vi "LaunchProgressBar.vi"(4 "error in":errorcluster, 5 "Title":string, 6 "MaxRange":i32) -> (0 "error out":errorcluster, 3 "reference out":refnum<vi>)   [LabVIEW 2018]
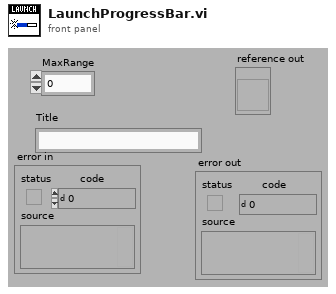
[diagram p1: front panel]
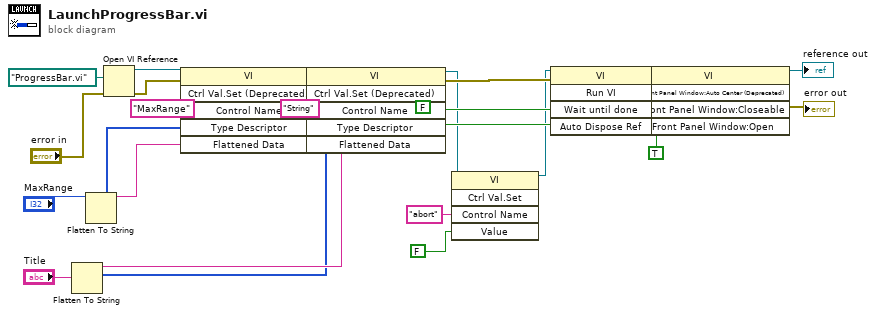
[diagram p0: block diagram]
diagram:
  w5 = FALSE ("Wait until done")
  w23 = TRUE
  n1 = Flatten To String(anything="Title") -> (data string=w12:string, type string=w11:i16[])  [unwired: 3 in, 1 out]
  n2 = Flatten To String(anything="MaxRange") -> (data string=w17:string, type string=w18:i16[])  [unwired: 3 in, 1 out]
  n3 = Open VI Reference(vi path=path "ProgressBar.vi", error in (no error)="error in") -> (vi reference=w20:refnum<vi>, error out=w15:errorcluster)  [unwired: 4 in]
  n4 = invoke class="VI" method="Ctrl Val.Set (Deprecated)"(reference=w20, error in=w15, "Control Name"="MaxRange", "Type Descriptor"=w18, "Flattened Data"=w17) -> (reference out=w14:refnum<vi>, error out=w13:errorcluster)  [unwired: 1 in, 4 out]
  n5 = invoke class="VI" method="Ctrl Val.Set (Deprecated)"(reference=w14, error in=w13, "Control Name"="String", "Type Descriptor"=w11, "Flattened Data"=w12) -> (reference out=w4:refnum<vi>, error out=w8:errorcluster)  [unwired: 1 in, 4 out]
  n6 = invoke class="VI" method="Ctrl Val.Set"(reference=w4, "Control Name"="abort", "Value"=FALSE) -> (reference out=w3:refnum<vi>)  [unwired: 2 in, 4 out]
  n7 = invoke class="VI" method="Run VI"(reference=w3, error in=w8, "Wait until done"=w5, "Auto Dispose Ref"=w5) -> (reference out=w6:refnum<vi>, error out=w7:errorcluster)  [unwired: 1 in, 3 out]
  n8 = property class="VI"(reference=w6, error in=w7, "Front Panel Window:Auto Center (Deprecated)"=w23, "Front Panel Window:Closeable"=w23, "Front Panel Window:Open"=w23) -> (reference out=→"reference out":refnum<vi>, error out=→"error out":errorcluster)
